vi "Ejercicio_2_2.vi"() -> ()   [LabVIEW 2020]
uses:
  <vilib>/numeric/Random Number (Range) DBL.vi
panel:
  out "min value":dbl
  out "max value":dbl
  out "EMA":dbl[](array[numeric])
  out "appended array":dbl[][](array[numeric])
  out "F°":dbl[](array[numeric])
  out "Datos obtenidos":dbl(graph)
  out "C°":dbl[](array[numeric])
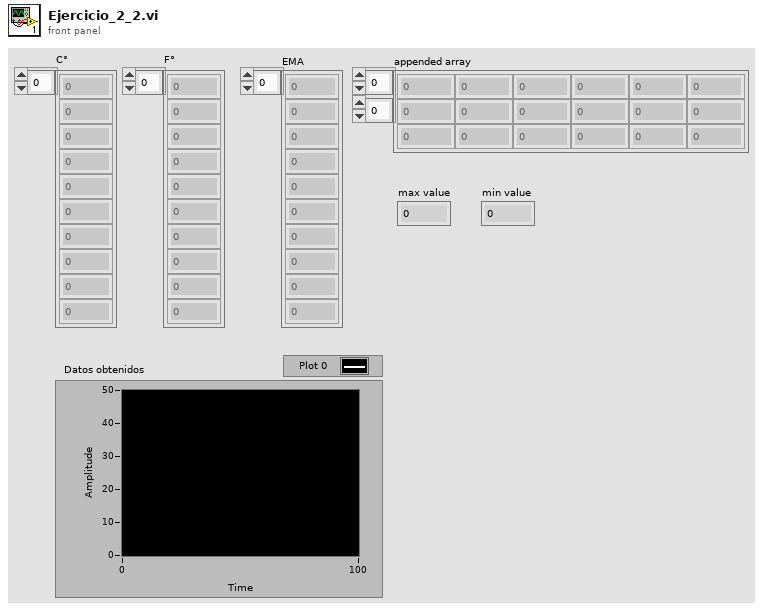
[diagram p1: front panel]
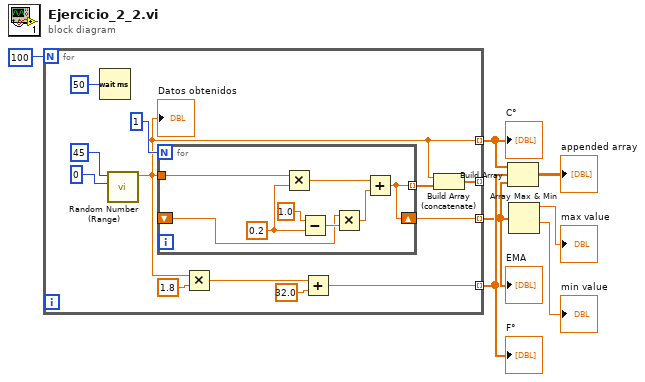
[diagram p0: block diagram]
diagram:
  n1 = for {
    N: 100 -> [_]
    tunnel: [w10] -> w4 mode=indexing
    tunnel: [w14] -> w6 mode=indexing
    tunnel: [w12] -> w3 mode=indexing
    tunnel: [w9] -> _ mode=indexing
    n2 = Wait (ms)(milliseconds to wait=u32 50) -> ()  [unwired: 1 out]
    n3 = call-poly <vilib>:"Random Number (Range).vi"("lower bound (0)"=u64 0, "upper bound (100)"=u64 45) -> ("number"=w10:dbl)  [unwired: 9 in]
    "Datos obtenidos" <- w10
    n4 = for {
      N: 1 -> [_]
      tunnel: w10 -> [w22]
      shift-right: [w20] -> w12
      shift-left: _ -> [w21]
      tunnel: [w20] -> w11 mode=indexing
      w24 = 0.2 ("y")
      n5 = Multiply(x=w22, y=w24) -> (x*y=w27:dbl)
      n6 = Subtract(x=1.0, y=w24) -> (x-y=w26:dbl)
      n7 = Multiply(x=w21, y=w26) -> (x*y=w23:dbl)
      n8 = Add(x=w27, y=w23) -> (x+y=w20:dbl)
    }
    n9 = Multiply(x=w10, y=1.8) -> (x*y=w19:dbl)
    n10 = Add(x=w19, y=32.0) -> (x+y=w14:dbl)
    n11 = Build Array (concatenate)(w10, w11) -> (w9:dbl[])
  }
  "C°" <- w4
  "F°" <- w6
  "EMA" <- w3
  n12 = Build Array(w4, w6, w3) -> (→"appended array":dbl[][])
  n13 = Array Max & Min(array=w3) -> (max value=→"max value":dbl, min value=→"min value":dbl)  [unwired: 2 out]
